vi "PID In Range_Buffer_Bool_VIG.vi"(7 "Operation":enum16{"get data", "set data", "initialize"}(ring)=enum."set data", 8 "error in":errorcluster, 9 "Current":bool, 11 "Boolean":bool) -> (0 "error out":errorcluster, 1 "Current in tol?":bool, 3 "Boolean 2":bool)   [LabVIEW 2018]
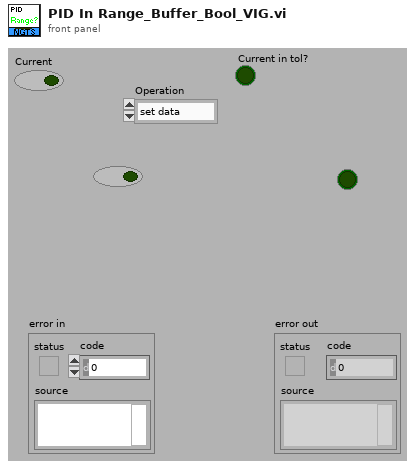
[diagram p1: front panel]
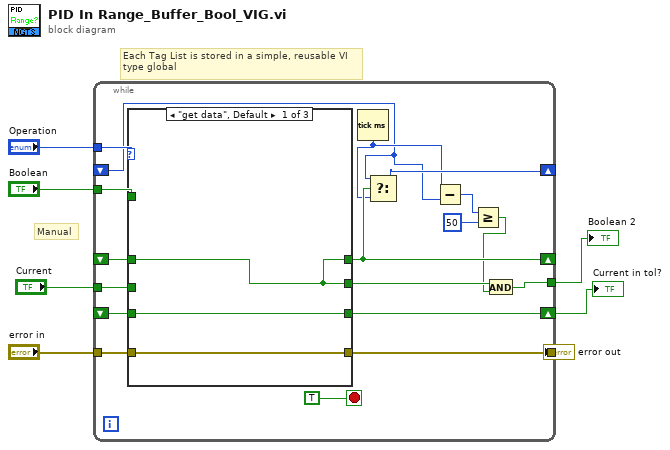
[diagram p0: block diagram]
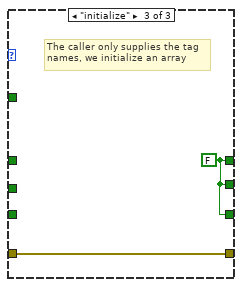
[diagram p3: hidden frame]
diagram:
  # "Manual"
  # "Each Tag List is stored in a simple, reusable VI\ntype global"
  n1 = while {
    tunnel: "Operation" -> [w25]
    tunnel: "Boolean" -> [w23]
    tunnel: "error in" -> [w22]
    tunnel: [w21] -> w5
    shift-right: [w18] -> _
    shift-left: _ -> [w20]
    tunnel: [w13] -> w4
    shift-right: [w17] -> _
    shift-left: _ -> [w15]
    shift-right: [w11] -> w3
    shift-left: _ -> [w10]
    tunnel: "Current" -> [w9]
    stop <- TRUE stop-if-true
    n2 = case shown="\"get data\", Default" w25 {
      tunnel: w23 -> [_ w30 _]
      tunnel: w22 -> [w28 w31 w33]
      tunnel: [w28 w31 w33] -> w21
      tunnel: [w27 w30 w32] -> w18
      tunnel: w20 -> [w27 _ _]
      tunnel: [w27 w30 w32] -> w19
      tunnel: [w26 w29 w32] -> w11
      tunnel: w10 -> [w26 _ _]
      tunnel: w9 -> [_ w29 _]
      frame "get data", Default {
      }
      frame "set data" {
      }
      frame "initialize" {
        w32 = FALSE ("Boolean")
        # "The caller only supplies the tag\nnames, we initialize an array"
      }
    }
    n3 = Tick Count (ms)() -> (millisecond timer value=w16:u32)
    n4 = Select(t=w15, s=w18, f=w16) -> (s? t:f=w17:u32)
    n5 = Subtract(x=w16, y=w15) -> (x-y=w14:u32)
    n6 = Greater Or Equal?(x=w14, y=u32 50) -> (x >= y?=w12:bool)
    n7 = And(x=w19, y=w12) -> (x .and. y?=w13:bool)
  }
  "error out" <- w5
  "Boolean 2" <- w4
  "Current in tol?" <- w3
